vi "Joystick test code_2.vi"() -> ()   [LabVIEW 2015]
uses:
  <vilib>/Utility/inputDevices.llb/joystickAcquire.vi
  <resource>/lvinput.dll
panel:
  in  "s":bool
  in  "Close":bool
  out "error out 2":errorcluster
  out "axis info 2":T1
  out "Read Error":errorcluster
  in  "Read":bool
  out "error out":errorcluster
  in  "Open":bool
  out "*(type *) &x 2":i32
  out "joystick info":T2(array[cluster])
  in  "stop":bool
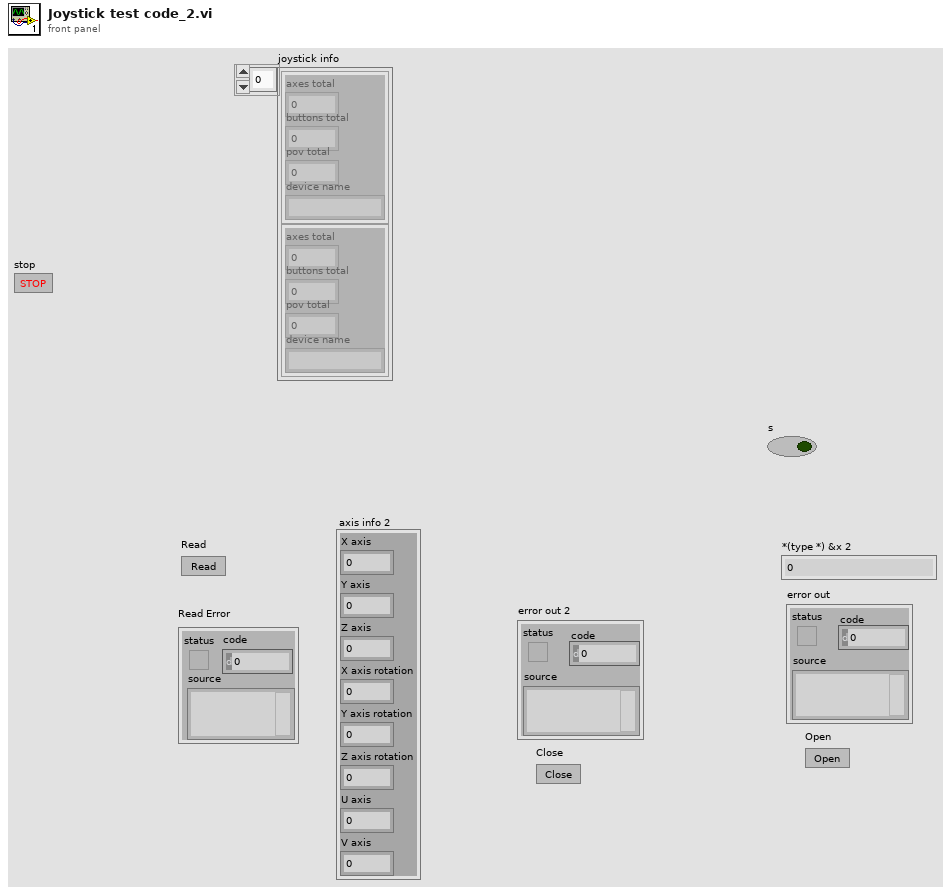
[diagram p1: front panel]
types:
  T1 = cluster{"X axis":i32, "Y axis":i32, "Z axis":i32, "X axis rotation":i32, "Y axis rotation":i32, "Z axis rotation":i32, "U axis":i32, "V axis":i32}
  T2 = cluster{"axes total":u32, "buttons total":u32, "pov total":u32, "device name":string}[]
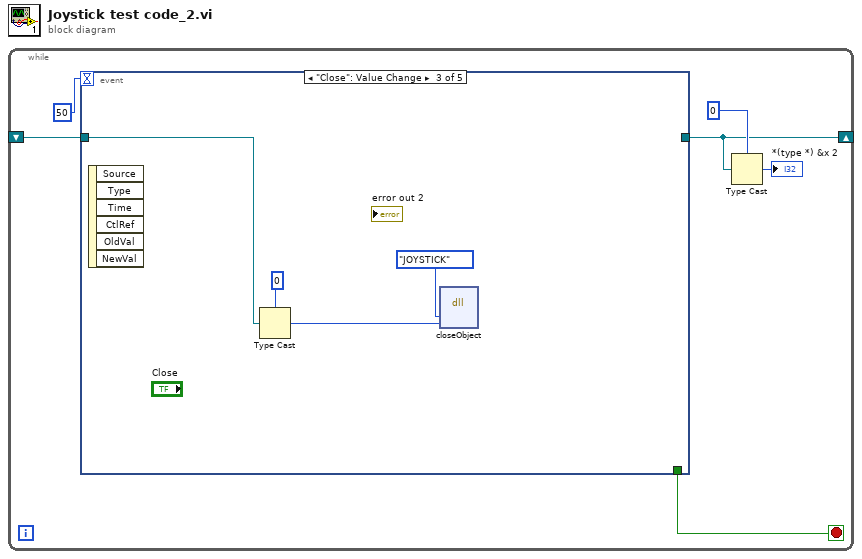
[diagram p0: block diagram]
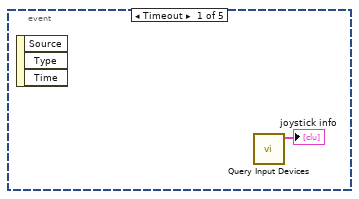
[diagram p2: hidden frame]
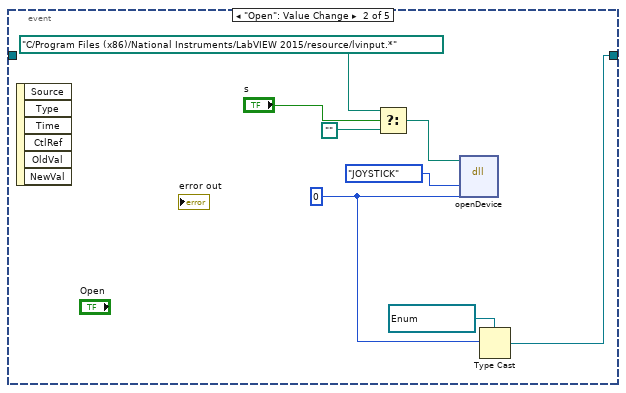
[diagram p3: hidden frame]
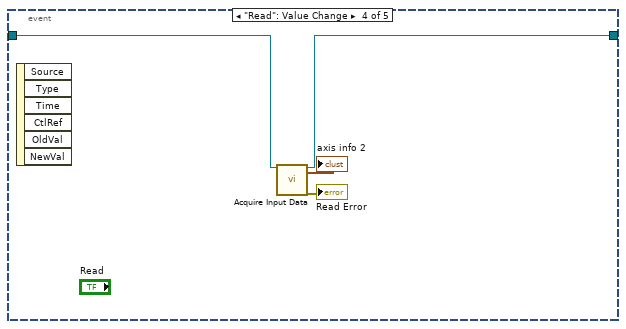
[diagram p4: hidden frame]
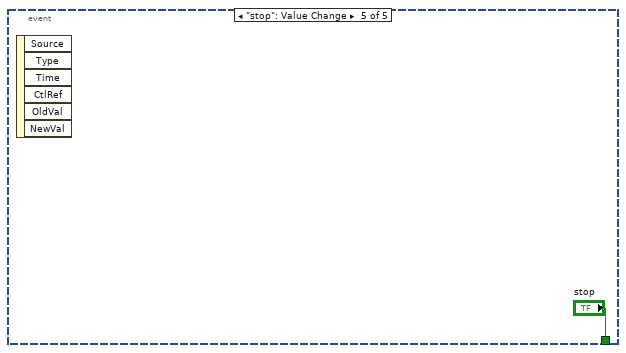
[diagram p5: hidden frame]
diagram:
  n1 = while {
    shift-right: [w1] -> _
    shift-left: _ -> [w4]
    stop <- w6 stop-if-true
    n2 = event shown="[2] \"Close\": Value Change" {
      selector: _ -> [_ _ _ _ _]
      dyn-events: _ -> [_ _ _ _ _]
      timeout: 50 -> [_ _ _ _ _]
      tunnel: [_ _ _ _ "stop"] -> w6
      tunnel: [_ w12 _ w20 _] -> w1
      tunnel: w4 -> [_ _ w16 w21 _]
      event Timeout {
        n3 = event-data() -> ()  [unwired: 1 in, 3 out]
        n4 = call <vilib>:"Query Input Devices.vi"() -> ("joystick info"=→"joystick info":T2)  [unwired: 8 in, 3 out]
      }
      event "Open": Value Change {
        w14 = refnum<k1> refnum items=["JOYSTICK"] ("JOYSTICK")
        w13 = 0 ("device index")
        n5 = event-data() -> ()  [unwired: 1 in, 6 out]
        n6 = Select(t=path "C:/Program Files (x86)/National Instruments/LabVIEW 2015/resource/lvinput.*" ("path in"), s="s", f=path "") -> (s? t:f=w10:path)
        n7 = dll-call lib="C:/Program Files (x86)/National Instruments/LabVIEW 2015/resource/lvinput.*" fn="openDevice"(path in=w10, enum16{"JOYSTICK", "KEYBOARD", "MOUSE"}."JOYSTICK" ("Enum"), w13) -> ()  [unwired: 5 in, 2 out]
        n8 = Type Cast(type=w14, x=w13) -> (*(type *) &x=w12:refnum<k1>)
      }
      event "Close": Value Change {
        n9 = event-data() -> ()  [unwired: 1 in, 6 out]
        n10 = Type Cast(type=0, x=w16) -> (*(type *) &x=w18:i32)
        n11 = dll-call lib="C:/Program Files (x86)/National Instruments/LabVIEW 2015/resource/lvinput.*" fn="closeObject"(enum16{"JOYSTICK", "KEYBOARD", "MOUSE"}."JOYSTICK" ("Enum"), w18) -> ()  [unwired: 6 in, 2 out]
      }
      event "Read": Value Change {
        n12 = event-data() -> ()  [unwired: 1 in, 6 out]
        n13 = call-poly <vilib>:"Acquire Input Data.vi"("device ID"=w21) -> ("device ID"=w20:refnum<k1>, "axis info"=→"axis info 2":T1, "error out"=→"Read Error":errorcluster)  [unwired: 14 in, 2 out]
      }
      event "stop": Value Change {
        n14 = event-data() -> ()  [unwired: 1 in, 6 out]
      }
    }
    n15 = Type Cast(type=0, x=w1) -> (*(type *) &x=→"*(type *) &x 2":i32)
  }
